vi "Broadcast Sensor Data.vi"(8 "error in (no error)":errorcluster, 10 "SensorData":refnum<class "SensorData.lvclass">, 11 "Sensor in":refnum<class "Sensor.lvclass">) -> (0 "error out":errorcluster, 3 "Sensor out":refnum<class "Sensor.lvclass">)   [LabVIEW 2012, in "Sensor Definition.lvlib" / "Sensor.lvclass"]
uses:
  Sensor.lvclass
  SensorData.lvclass
  Sensor.lvclass/Sensor.ctl
  <vilib>/ActorFramework/Message Enqueuer/Message Priority.ctl
  SensorView Messages/Update Sensor Data Msg/Update Sensor Data Msg.lvclass/Update Sensor Data Msg.ctl
  <vilib>/ActorFramework/Message Enqueuer/Message Enqueuer.lvclass/Message Enqueuer.ctl
  Read Listening SensorViews.vi
  <vilib>/ActorFramework/Message Enqueuer/Enqueue.vi
  <vilib>/ActorFramework/Message Priority Queue/Priority Enqueue.vi
  <vilib>/ActorFramework/Message Enqueuer/Message Enqueuer.lvclass
  SensorView Messages/Update Sensor Data Msg/Update Sensor Data Msg.lvclass
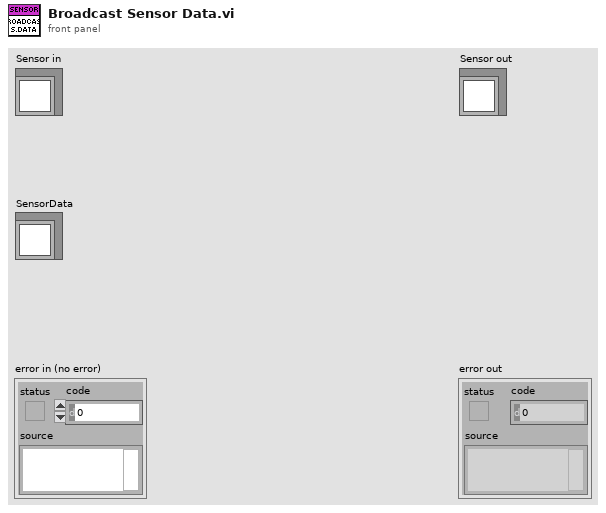
[diagram p1: front panel]
types:
  T1 = typedef "Actor Framework.lvlib/Message Enqueuer.lvclass/Message Priority.ctl" = enum16{"Low", "Normal", "High"}
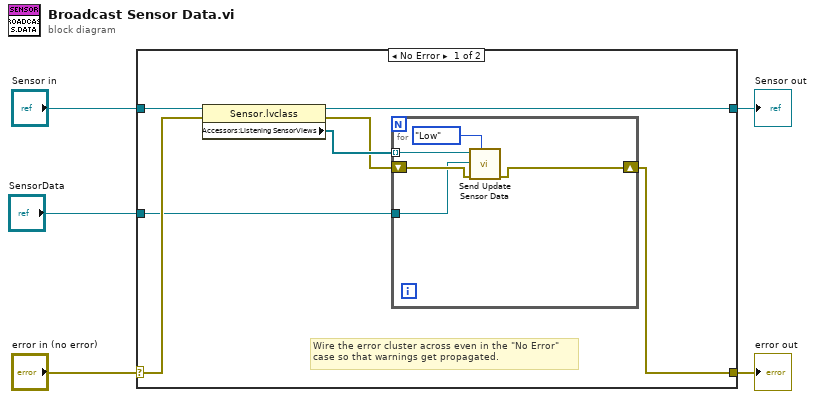
[diagram p0: block diagram]
diagram:
  n1 = case shown="No Error" "error in (no error)" {
    selector: "error in (no error)" -> [w8 w19]
    tunnel: [w7 w19] -> w4
    tunnel: [w11 w18] -> w2
    tunnel: "Sensor in" -> [w12 w18]
    tunnel: "SensorData" -> [w6 _]
    frame No Error {
      # "Wire the error cluster across even in the \"No Error\"\ncase so that warnings get propagated."
      n2 = property class="Sensor.lvclass"(reference=w12, error in=w8) -> (reference out=w11:refnum<class "Sensor.lvclass">, error out=w9:errorcluster, "Accessors:Listening SensorViews"=w10:refnum<class "Message Enqueuer.lvclass">[])
      n3 = for {
        tunnel: w10 -> [w17] mode=indexing
        shift-right: [w15] -> w7
        shift-left: w9 -> [w16]
        tunnel: w6 -> [w14]
        n4 = call "Send Update Sensor Data.vi"("Message Priority (Normal)"=Message_Priority."Low", "error in (no error)"=w16, "SensorData"=w14, "Message Enqueuer"=w17) -> ("error out"=w15:errorcluster)  [unwired: 6 in, 1 out]
      }
    }
    frame Error {
    }
  }
  "error out" <- w4
  "Sensor out" <- w2
